vi "init.vi"(8 "error in":errorcluster, 10 "TBM module configuration in":refnum<class "TBM module configuration.lvclass">, 11 "PID Module 2 runtime in":refnum<class "PID Module 2 runtime.lvclass">) -> (0 "error out":errorcluster, 1 "data allocations":T1, 2 "execution settings":T4, 3 "PID Module 2 runtime out":refnum<class "PID Module 2 runtime.lvclass">)   [LabVIEW 2015, in "PID Module 2 runtime.lvclass"]
doc: "Provides an interface for initializing a module at runtime. While this interface performs no operations, a child should provide an override which may open any necessary references or sessions, allocate necessary memory, and perform any final configuration validataion before providing the full configuration <b>execution data</b> to the calling process."
uses:
  PID Module 2 runtime.lvclass
  <vilib>/NI/Tag Bus Module Framework/module configuration/TBM module configuration.lvclass
  <vilib>/NI/Tag Bus Module Framework/runtime/execution settings.ctl
  <vilib>/NI/Tag Bus Module Framework/channel/data tables.ctl
  <vilib>/NI/Tag Bus/dictionary/data dictionary.lvclass
  <vilib>/NI/Tag Bus/dictionary table pair.ctl
  <vilib>/NI/Tag Bus/table/data table.ctl
  configuration/PID Module 2 configuration.lvclass
  configuration/PID Module 2 configuration.lvclass/PID Module 2 configuration.ctl
  PID Module 2 runtime.lvclass/PID Module 2 runtime.ctl
  <vilib>/NI/Tag Bus Module Framework/channel/TBM channel.lvclass
  <vilib>/NI/Tag Bus Module Framework/runtime/TBM module execution interface.lvclass
  <vilib>/NI/Tag Bus/tag bus.lvlib
  <vilib>/NI/Tag Bus/table/data table.lvlib
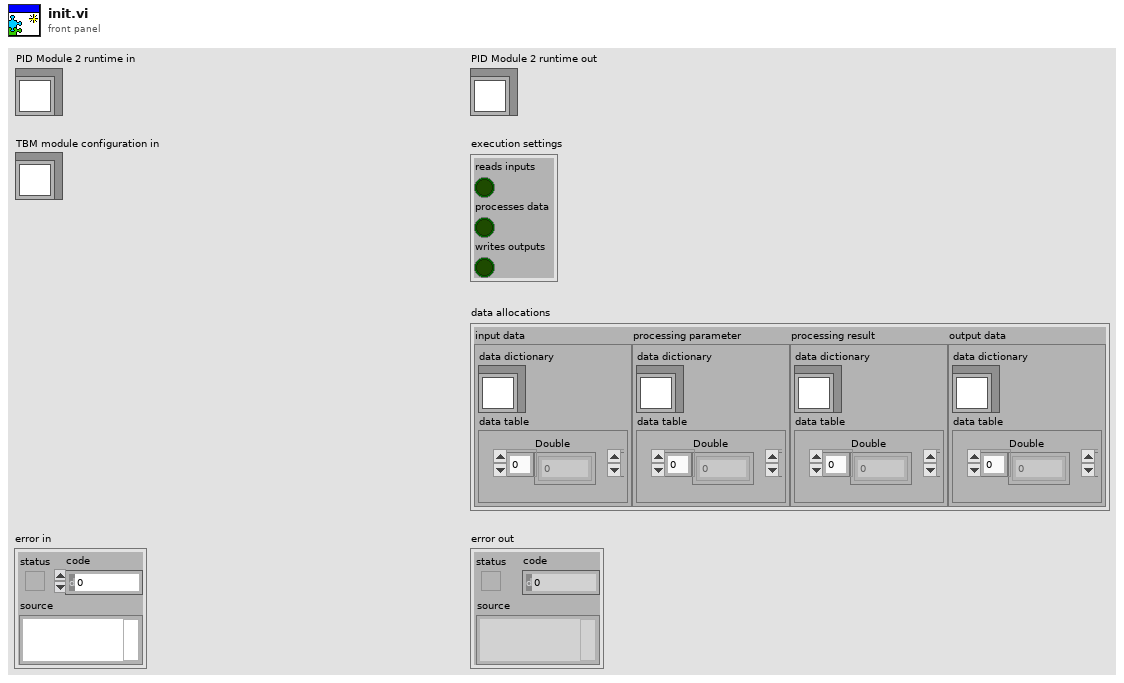
[diagram p1: front panel]
types:
  T1 = typedef "TBM channel.lvclass/data tables.ctl" = cluster{"input data":T2, "processing parameter":T2, "processing result":T2, "output data":T2}
  T2 = typedef "tag bus.lvlib/dictionary table pair.ctl" = cluster{"data dictionary":refnum<class "data dictionary.lvclass">, "data table":T3}
  T3 = typedef "tag bus.lvlib/data table.lvlib/data table.ctl" = cluster{"Double":dbl[], "Single":sgl[], "I64":i64[], "I32":i32[], "I16":i16[], "I8":i8[], "U64":u64[], "U32":u32[], "U16":u16[], "U8":u8[], "Boolean":bool[], "String":string[], "Array of Double":cluster{"DBL Array":dbl[]}[], "Array of Single":cluster{"SGL Array":sgl[]}[], "Array of I64":cluster{"I64 Array":i64[]}[], "Array of I32":cluster{"I32 Array":i32[]}[], "Array of I16":cluster{"I16 Array":i16[]}[], "Array of I8":cluster{"I8 Array":i8[]}[], "Array of U64":cluster{"U64 Array":u64[]}[], "Array of U32":cluster{"U32 Array":u32[]}[], "Array of U16":cluster{"U16 Array":u16[]}[], "Array of U8":cluster{"U8 Array":u8[]}[], "Array of Boolean":cluster{"Boolean Array":bool[]}[], "Array of String":cluster{"String Array":string[]}[]}
  T4 = typedef "TBM module execution interface.lvclass/execution settings.ctl" = cluster{"reads inputs":bool, "processes data":bool, "writes outputs":bool}
  T5 = typedef "PID Module 2 configuration.lvclass/Line.ctl" = cluster{"PID ID":string, "Setpoint":refnum<class "TBM channel.lvclass">, "Variable":refnum<class "TBM channel.lvclass">, "Output":refnum<class "TBM channel.lvclass">, "Output High":refnum<class "TBM channel.lvclass">, "Output Low":refnum<class "TBM channel.lvclass">, "P":refnum<class "TBM channel.lvclass">, "I":refnum<class "TBM channel.lvclass">, "D":refnum<class "TBM channel.lvclass">}
  T6 = typedef "PID Module 2 runtime.lvclass/Mapping.ctl" = cluster{"Setpoints":i32[], "Variable":i32[], "Output":i32[], "High":i32[], "Low":i32[], "P":i32[], "I":i32[], "D":i32[]}
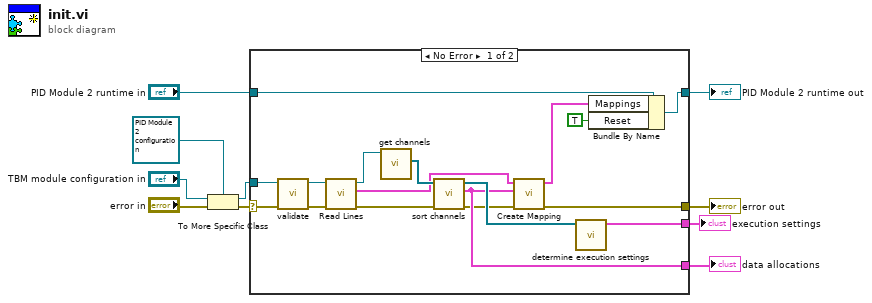
[diagram p0: block diagram]
diagram:
  n1 = To More Specific Class(target class=refnum<class "PID Module 2 configuration.lvclass"> refnum ("Synchronous module configuration"), reference="TBM module configuration in", error in="error in") -> (specific class reference=w9:refnum<class "PID Module 2 configuration.lvclass">, error out=w10:errorcluster)
  n2 = case shown="No Error" w10 {
    selector: w10 -> [w25 w28]
    tunnel: w9 -> [w24 _]
    tunnel: "PID Module 2 runtime in" -> [w20 w29]
    tunnel: [w19 w29] -> w4
    tunnel: [w15 w28] -> w3
    tunnel: [w21 _] -> w1
    tunnel: [w27 _] -> w2
    frame No Error {
      n3 = call-dynamic "validate.vi"("error in"=w25, "PID Module 2 configuration in"=w24) -> ("error out"=w14:errorcluster, "PID Module 2 configuration out"=w12:refnum<class "PID Module 2 configuration.lvclass">)  [unwired: 8 in]
      n4 = call "Read Lines.vi"("error in (no error)"=w14, "PID Module 2 configuration in"=w12) -> ("error out"=w13:errorcluster, "Lines"=w22:T5[], "PID Module 2 configuration out"=w11:refnum<class "PID Module 2 configuration.lvclass">)  [unwired: 7 in]
      n5 = call-dynamic "get channels.vi"("PID Module 2 configuration in"=w11) -> ("channels"=w23:refnum<class "TBM channel.lvclass">[])  [unwired: 9 in, 1 out]
      n6 = call <vilib>:"sort channels.vi"("error in"=w13, "channels in"=w23) -> ("error out"=w16:errorcluster, "data allocations"=w21:T1, "channels out"=w26:refnum<class "TBM channel.lvclass">[])  [unwired: 7 in]
      n7 = call "Create Mapping.vi"("error in (no error)"=w16, "data allocations"=w21, "Lines"=w22) -> ("error out"=w15:errorcluster, "Mappings"=w17:T6)  [unwired: 7 in]
      n8 = call <vilib>:"determine execution settings.vi"("channels"=w26) -> ("execution settings"=w27:T4)  [unwired: 10 in]
      n9 = Bundle By Name(cluster=w20, "Mappings"=w17, "Reset"=TRUE) -> (w19:refnum<class "PID Module 2 runtime.lvclass">)
    }
    frame Error {
    }
  }
  "error out" <- w3
  "PID Module 2 runtime out" <- w4
  "execution settings" <- w2
  "data allocations" <- w1
